vi "Top Level Launcher.vi"(6 "Variant in":variant, 7 "Shift Pressed?":bool, 8 "error in":errorcluster, 10 "QD Combo Box Ref":refnum<vi>, 11 "QD Launch VI Ref":refnum<vi>) -> (0 "error out":errorcluster, 4 "Variant out":variant)   [LabVIEW 2020]
doc: "Sets or run the top level VI in the project.\n\nNormal Operation:\nTo set the top VI, use Shift+Ctrl+[shortcut].\nTo run the top VI, use Ctrl+[shortcut].\n\nAdvanced Operation using QD data entry:\nTo set the top VI, enter \"s\" or \"set\" before activating the shortcut.\nTo run the top VI, enter \"r\" or \"run\" before activating the shortcut.\nTo remove the top VI setting, enter \"d\", \"del\", \"delete\", \"rem\", or \"remove\" before activating the shortcut.\nTo read what the top VI is, enter \"get\" or \"read\" before activating the shortcut.\n\nDefault Shortcut - [E]"
panel:
  in  "Undo Name":string="Quick Drop Keyboard Shortcut"
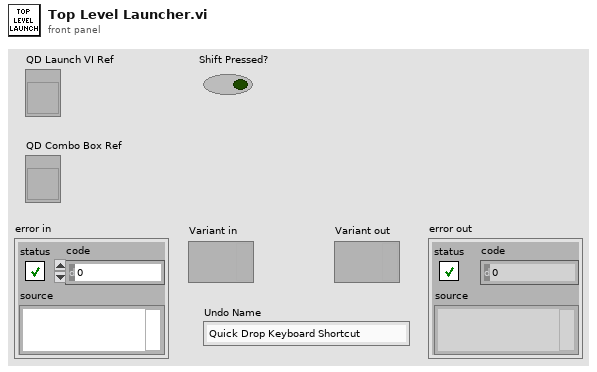
[diagram p1: front panel]
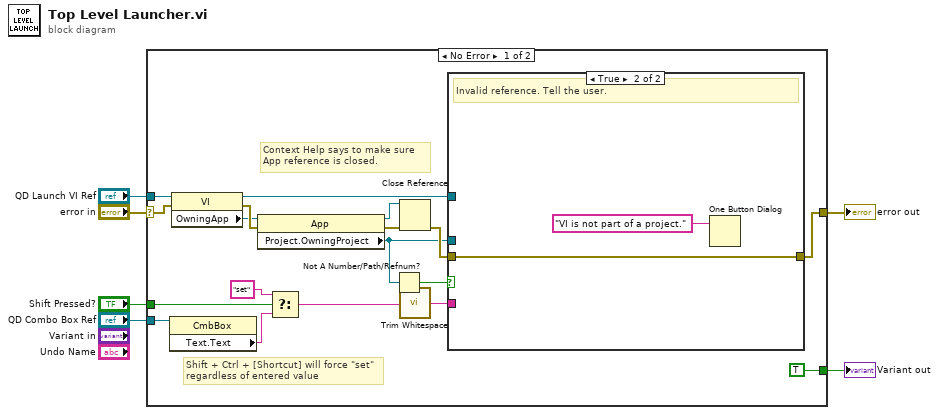
[diagram p0: block diagram]
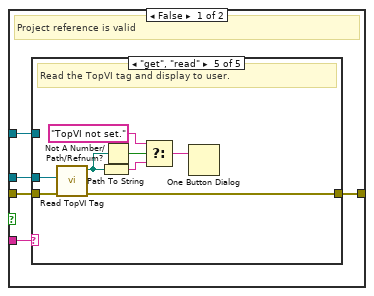
[diagram p2: hidden frame]
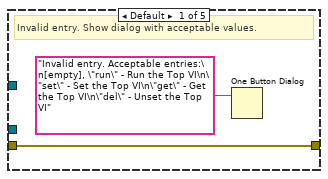
[diagram p3: hidden frame]
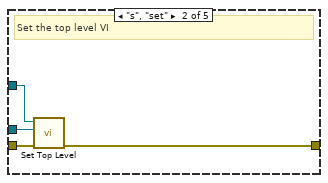
[diagram p4: hidden frame]
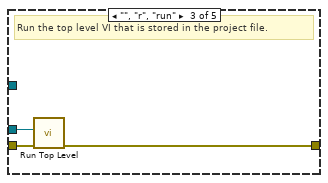
[diagram p5: hidden frame]
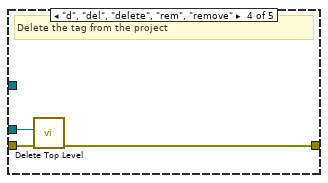
[diagram p6: hidden frame]
diagram:
  n1 = case shown="No Error" "error in" {
    selector: "error in" -> [w23 w52]
    tunnel: [w24 w52] -> w5
    tunnel: "QD Launch VI Ref" -> [w8 _]
    tunnel: "Shift Pressed?" -> [w18 _]
    tunnel: [TRUE _] -> w2
    tunnel: "QD Combo Box Ref" -> [w12 _]
    frame No Error {
      # "Context Help says to make sure App reference is closed."
      # "Shift + Ctrl + [Shortcut] will force \"set\"\nregardless of entered value"
      n2 = property class="CmbBox"(reference=w12) -> ("Text.Text"=w11:string)  [unwired: 1 in, 2 out]
      n3 = property class="VI"(reference=w8, error in=w23) -> (reference out=w9:refnum<vi>, error out=w22:errorcluster, "OwningApp"=w10:refnum<vi>)
      n4 = property class="App"(reference=w10, error in=w22) -> (reference out=w7:refnum<vi>, error out=w21:errorcluster, "Project.OwningProject"=w14:refnum<vi>)
      n5 = Select(t="set", s=w18, f=w11) -> (s? t:f=w16:string)
      n6 = Not A Number/Path/Refnum?(number/path/refnum=w14) -> (NaN/Path/Refnum?=w15:bool)
      n7 = Close Reference(reference=w7, error in (no error)=w21) -> (error out=w20:errorcluster)
      n8 = call <vilib>:"Trim Whitespace.vi"("string"=w16) -> ("trimmed string"=w13:string)  [unwired: 1 in]
      n9 = case shown="True" w15 {
        tunnel: w13 -> [w27 _]
        tunnel: [w29 w51] -> w24
        tunnel: w20 -> [w28 w51]
        tunnel: w9 -> [w26 _]
        tunnel: w14 -> [w25 _]
        frame False {
          # "Project reference is valid"
          n10 = case shown="\"get\", \"read\"" w27 {
            tunnel: w28 -> [w31 w35 w38 w41 w49]
            tunnel: [w31 w34 w37 w40 w48] -> w29
            tunnel: w26 -> [_ w33 _ _ _]
            tunnel: w25 -> [_ w32 w36 w39 w47]
            frame Default {
              # "Invalid entry. Show dialog with acceptable values."
              n11 = One Button Dialog(message="Invalid entry. Acceptable entries:\n[empty], \"run\" - Run the Top VI\n\"set\" - Set the Top VI\n\"get\" - Get the Top VI\n\"del\" - Unset the Top VI") -> ()  [unwired: 1 in, 1 out]
            }
            frame "s", "set" {
              # "Set the top level VI"
              n12 = call "Set Top Level.vi"("error in"=w35, "Project Reference"=w32, "VI Reference"=w33) -> ("error out"=w34:errorcluster)  [unwired: 8 in]
            }
            frame "", "r", "run" {
              # "Run the top level VI that is stored in the project file."
              n13 = call "Run Top Level.vi"("error in"=w38, "Project Reference"=w36) -> ("error out"=w37:errorcluster)  [unwired: 9 in]
            }
            frame "d", "del", "delete", "rem", "remove" {
              # "Delete the tag from the project"
              n14 = call "Delete Top Level.vi"("error in"=w41, "Project Reference"=w39) -> ("error out"=w40:errorcluster)  [unwired: 9 in]
            }
            frame "get", "read" {
              # "Read the TopVI tag and display to user."
              n15 = call "Read TopVI Tag.vi"("error in"=w49, "Project Reference"=w47) -> ("error out"=w48:errorcluster, "TopVI Path"=w46:path)  [unwired: 7 in, 1 out]
              n16 = Path To String(path=w46) -> (string=w44:string)
              n17 = Not A Number/Path/Refnum?(number/path/refnum=w46) -> (NaN/Path/Refnum?=w45:bool)
              n18 = Select(t="TopVI not set.", s=w45, f=w44) -> (s? t:f=w42:string)
              n19 = One Button Dialog(message=w42) -> ()  [unwired: 1 in, 1 out]
            }
          }
        }
        frame True {
          # "Invalid reference. Tell the user."
          n20 = One Button Dialog(message="VI is not part of a project.") -> ()  [unwired: 1 in, 1 out]
        }
      }
    }
    frame Error {
    }
  }
  "error out" <- w5
  "Variant out" <- w2
